vi "CODCr质控流程 (子VI).vi"(10 "CODCr量程切换":enum32{"H", "L", "AUTO"}(ring)=enum."AUTO", 11 "CODCr":bool) -> (2 "CODCr中断报警":bool, 3 "布尔":bool)   [LabVIEW 2016, in "质控单元.lvlib"]
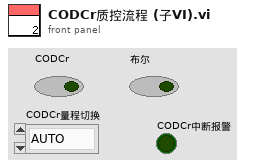
[diagram p1: front panel]
types:
  T1 = enum16{"待机", "启动水样测量", "水样测量中", "启动加标", "启动加标回收", "加标回收测量中", "结束"}
  T2 = cluster{"测量模式":enum16{"水样测量", "标样核查", "零点核查", "跨度核查", "空白测试", "加标回收", "平行样", "校零", "校标"}}
  T3 = enum16{"空闲", "水样测试", "标样核查", "零点核查", "跨度核查", "空白测试", "平行样测试", "加标回收", "空白校准", "标样校准", "初始化（清洗）"}
  T4 = cluster{"系统时间":timestamp, "工作状态":enum16{"空闲", "水样测试", "标样核查", "零点核查", "跨度核查", "空白测试", "平行样测试", "加标回收", "空白校准", "标样校准", "初始化（清洗）"}, "测量模式":enum16{"待机", "连续模式", "周期模式", "定点模式", "受控模式", "手动模式"}, "告警代码":enum16{"无告警", "缺试剂告警", "缺水样告警", "缺蒸馏水告警", "缺标液告警", "仪表漏液告警", "标定异常告警", "超量程告警", "加热异常", "低试剂预警", "超上限告警", "超下限告警", "仪表内部其他异常", "滴定异常告警", "电极异常告警", "量程切换告警", "参数设置告警", "PH电极电位异常", "电导率电极异常", "浊度光度异常", "溶解氧电极异常", "溶解氧光强异常", "温度异常告警", "PH异常告警", "溶解氧异常告警", "电导率异常告警", "浊度异常告警", "叶绿素异常告警", "藻密度异常告警", "蓝绿藻异常告警", "ORP异常告警", "氨氮异常告警", "清洁刷异常告警", "SD卡异常告警", "蓝牙异常告警", "Wifi异常告警", "流程异常告警"}, "故障代码":enum16{"无故障", "电机故障", "温度故障", "通讯故障", "滴定故障"}, "日志代码":u16, "软件版本":u16, "F0":sgl, "F1":sgl, "F2":sgl, "F3":sgl, "T":sgl, "H":sgl, "id":u16, "flowid":u16, "量程":u16, "总磷控温温度1":sgl, "营养盐控温温度2":sgl, "ADC":sgl}
  T5 = cluster{"因子编码":u32, "单位":u16, "标样参考值":sgl, "水样数据时间":timestamp, "水样实测值":sgl, "水样数据标识":string, "标样数据时间":timestamp, "标样实测值":sgl, "标样数据标识":string, "空白数据时间":timestamp, "空白实测值":sgl, "空白数据标识":string, "零点核查数据时间":timestamp, "零点核查实测值":sgl, "零点核查数据标识":string, "跨度核查数据时间":timestamp, "跨度核查实测值":sgl, "跨度核查数据标识":string, "加标回收数据时间":timestamp, "加标回收实测值":sgl, "加标回收数据标识":string, "平行样数据时间":timestamp, "平行样实测值":sgl, "平行样数据标识":string}
  T6 = cluster{"量程":dbl, "检出限":dbl, "加标前水样浓度":dbl, "加标后水样浓度":dbl, "加标水杯定容体积":dbl, "加标母液浓度":dbl, "加标体积":dbl, "加标回收率":dbl}
  T7 = cluster{"氨氮":u8, "总磷":u8, "总氮":u8, "CODMn":u8, "CODCr":u8}
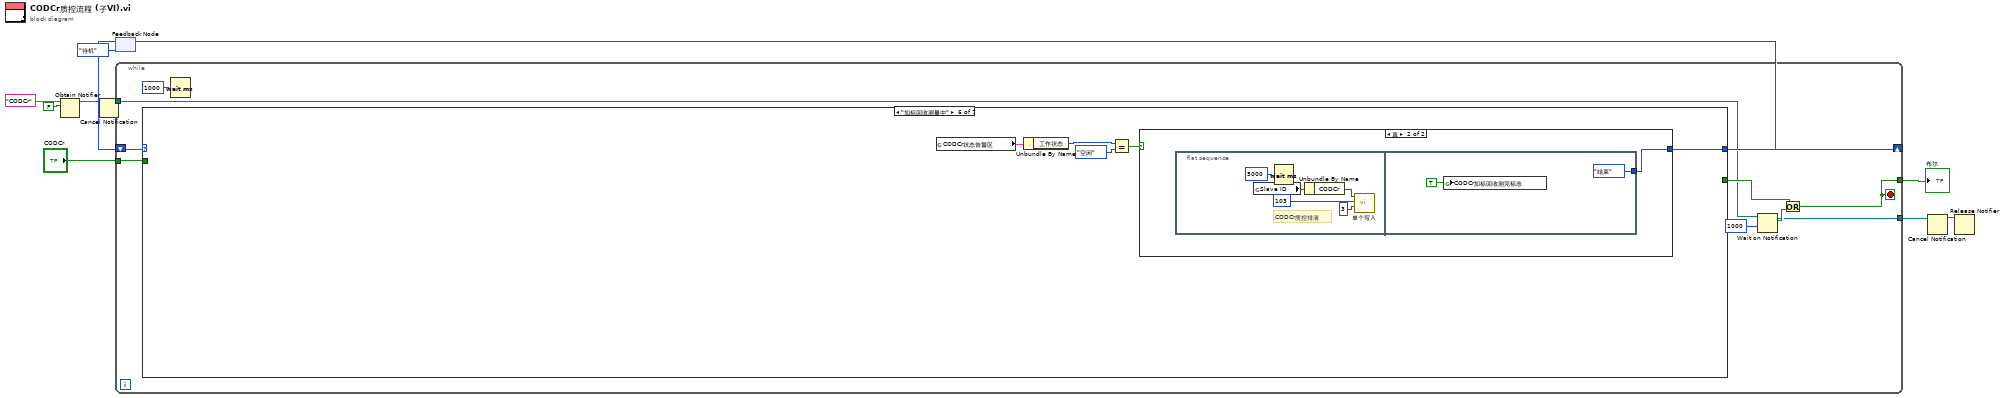
[diagram p0: block diagram]
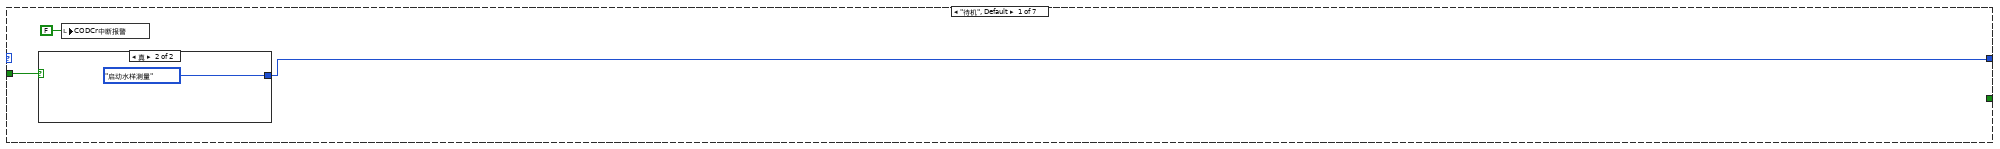
[diagram p2: hidden frame]
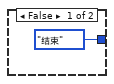
[diagram p3: hidden frame]
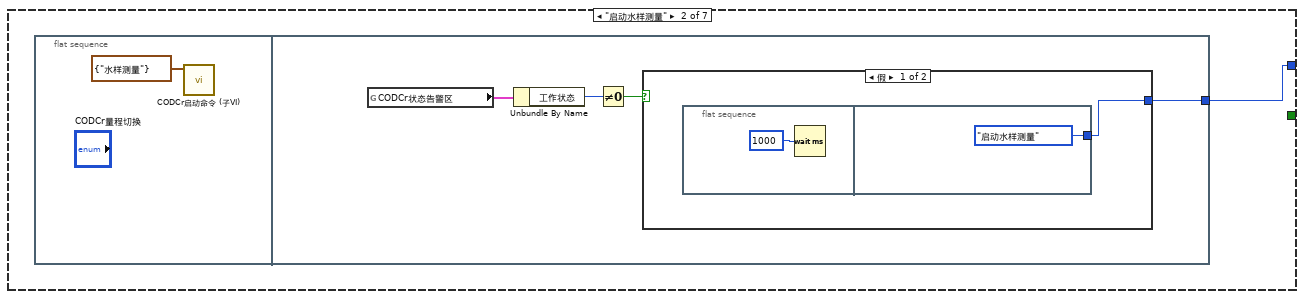
[diagram p4: hidden frame]
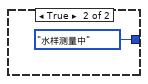
[diagram p5: hidden frame]
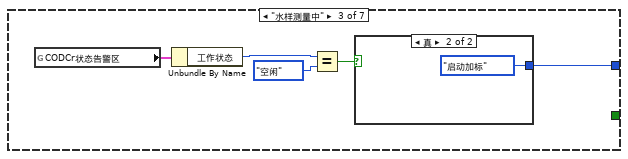
[diagram p6: hidden frame]
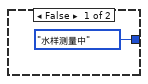
[diagram p7: hidden frame]
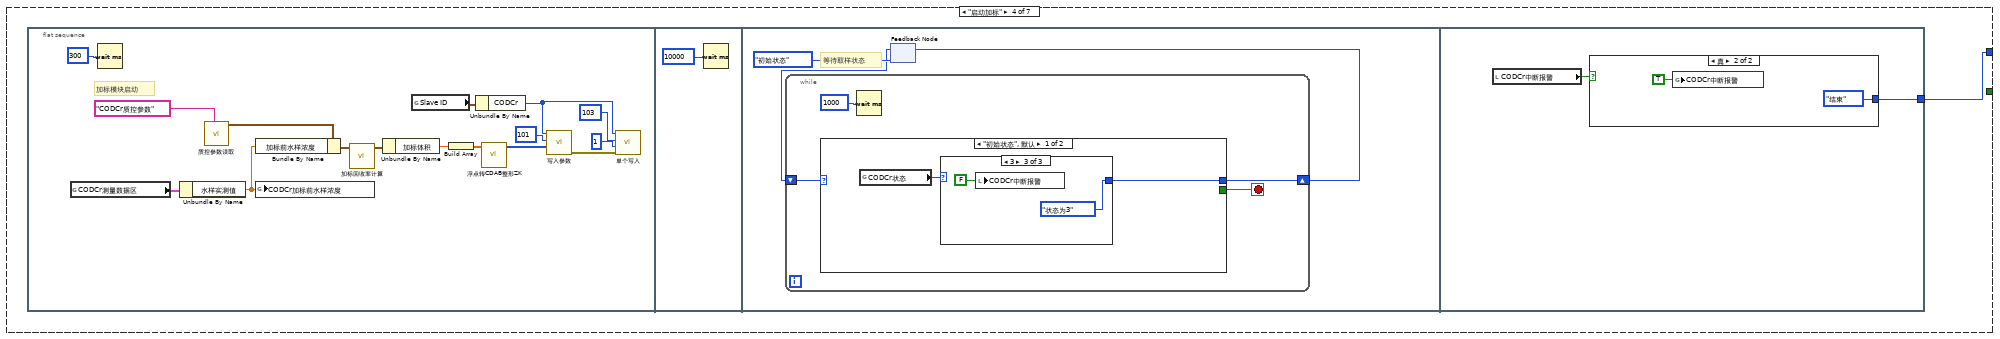
[diagram p8: hidden frame]
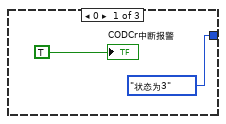
[diagram p9: hidden frame]
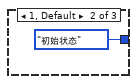
[diagram p10: hidden frame]
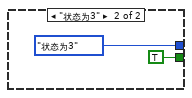
[diagram p11: hidden frame]
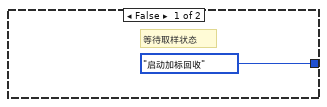
[diagram p12: hidden frame]
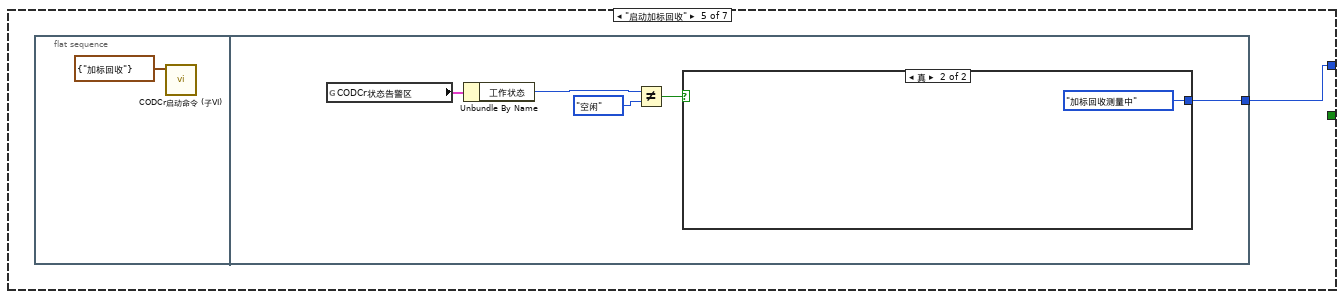
[diagram p13: hidden frame]
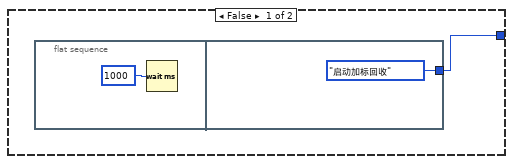
[diagram p14: hidden frame]
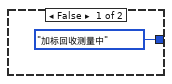
[diagram p15: hidden frame]
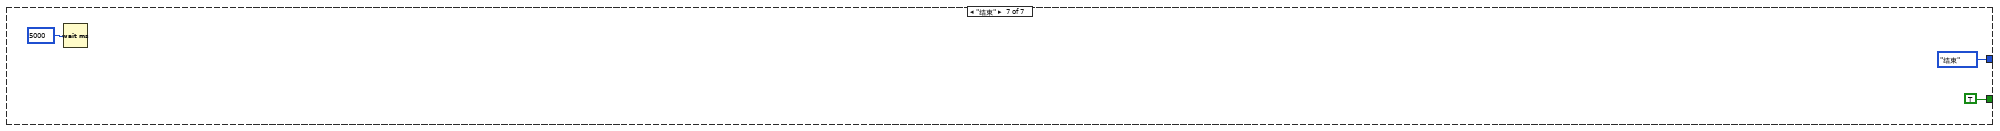
[diagram p16: hidden frame]
diagram:
  n1 = Obtain Notifier(name (unnamed)="CODCr" ("名称（未命名）"), notification data type=FALSE) -> (notifier out=w2:refnum<notifier>)  [unwired: 2 in, 2 out]
  n2 = Cancel Notification(0:w2) -> (8:w1:refnum<notifier>)  [unwired: 1 in, 2 out]
  n3 = feedback #1(T1."待机") -> (w7:T1)
  n4 = while {
    tunnel: "CODCr" -> [w21]
    tunnel: [w13] -> w9
    shift-right: [w20] -> w10
    shift-left: w7 -> [w18]
    tunnel: [w15] -> w3
    tunnel: w1 -> [w14]
    stop <- w13 stop-if-true
    n5 = case shown="\"加标回收测量中\"" w18 {
      tunnel: [w24 w27 w41 w44 w83 w98 T1."结束"] -> w20
      tunnel: [_ _ _ _ _ _ TRUE] -> w16
      tunnel: w21 -> [w23 _ _ _ _ _ _]
      frame "待机", Default {
        n6 = case shown="真" w23 {
          tunnel: [T1."结束" T1."启动水样测量"] -> w24
          frame False {
          }
          frame True {
          }
        }
        n7 = local write "CODCr中断报警"(FALSE ("CODMn中断报警")) -> ()
      }
      frame "启动水样测量" {
        n8 = flat-sequence {
          tunnel: [w32] -> w27
          frame #0 {
            n9 = call "CODCr启动命令 (子VI).vi"("启动测量模式"=T2 {"测量模式"=enum."水样测量"}) -> ()  [unwired: 10 in, 1 out]
          }
          frame #1 {
            n10 = global read "与CODCr交互全局.vi" "CODCr状态告警区"() -> (w30:T4)
            n11 = Unbundle By Name(w30) -> ("工作状态"=w31:T3)
            n12 = Not Equal To 0?(x=w31) -> (x != 0?=w29:bool)
            n13 = case shown="假" w29 {
              tunnel: [w33 T1."水样测量中"] -> w32
              frame False {
                n14 = flat-sequence {
                  tunnel: [T1."启动水样测量"] -> w33
                  frame #0 {
                    n15 = Wait (ms)(milliseconds to wait=u32 1000 ("等待时间（毫秒）")) -> ()  [unwired: 1 out]
                  }
                  frame #1 {
                  }
                }
              }
              frame True {
              }
            }
          }
        }
      }
      frame "水样测量中" {
        n16 = global read "与CODCr交互全局.vi" "CODCr状态告警区"() -> (w38:T4)
        n17 = Unbundle By Name(w38) -> ("工作状态"=w37:T3)
        n18 = Equal?(x=w37, y=T3."空闲") -> (x = y?=w39:bool)
        n19 = case shown="真" w39 {
          tunnel: [T1."水样测量中" T1."启动加标"] -> w41
          frame False {
          }
          frame True {
          }
        }
      }
      frame "启动加标" {
        n20 = flat-sequence {
          tunnel: [w79] -> w44
          frame #0 {
            # "加标模块启动"
            n21 = global read "与CODCr交互全局.vi" "CODCr测量数据区"() -> (w47:T5)
            n22 = Wait (ms)(milliseconds to wait=u32 300 ("等待时间（毫秒）")) -> ()  [unwired: 1 out]
            n23 = Unbundle By Name(w47) -> ("水样实测值"=w48:sgl)
            n24 = call "质控参数读取.vi"("section"="CODCr质控参数") -> ("参数"=w58:T6)  [unwired: 9 in, 1 out]
            n25 = Bundle By Name(cluster=w58, "加标前水样浓度"=w48) -> (w59:T6)
            n26 = global write "水样浓度全局.vi" "CODCr加标前水样浓度"(w48) -> ()
            n27 = call "加标回收率计算.vi"("参数"=w59) -> ("参数 out"=w57:T6)  [unwired: 9 in, 1 out]
            n28 = Unbundle By Name(w57) -> ("加标体积"=w50:dbl)
            n29 = global read "断电保存全局.vi" "Slave ID"() -> (w46:T7)
            n30 = Build Array(w50) -> (w56:dbl[])
            n31 = Unbundle By Name(w46) -> ("CODCr"=w45:u8)
            n32 = call "浮点转CDAB整形ZK.vi"("浮点数"=w56) -> ("CDAB整形输出"=w51:u16[])  [unwired: 10 in]
            n33 = call "写入参数.vi"("values"=w51, "starting address"=u16 101, "Slave ID"=w45) -> ("error out"=w55:errorcluster)  [unwired: 8 in]
            n34 = call "单个写入.vi"("Error in"=w55, "value"=u16 1, "address"=u16 103, "Slave ID"=w45) -> ()  [unwired: 7 in, 1 out]
          }
          frame #1 {
            n35 = Wait (ms)(milliseconds to wait=u32 10000 ("等待时间（毫秒）")) -> ()  [unwired: 1 out]
          }
          frame #2 {
            # "等待取样状态"
            n36 = feedback #2(enum16{"初始状态", "状态为3"}."初始状态") -> (w63:enum16{"初始状态", "状态为3"})
            n37 = while {
              shift-right: [w67] -> w62
              shift-left: w63 -> [w68]
              stop <- w66 stop-if-true
              n38 = case shown="\"初始状态\", 默认" w68 {
                tunnel: [w70 enum16{"初始状态", "状态为3"}."状态为3"] -> w67
                tunnel: [_ TRUE] -> w66
                frame "初始状态", Default {
                  n39 = global read "加标回收状态全局变量.vi" "CODCr状态"() -> (w69:u16)
                  n40 = case shown="3" w69 {
                    tunnel: [enum16{"初始状态", "状态为3"}."状态为3" enum16{"初始状态", "状态为3"}."初始状态" enum16{"初始状态", "状态为3"}."状态为3"] -> w70
                    frame 0 {
                      "CODCr中断报警" <- TRUE ("CODMn中断报警")
                    }
                    frame 1, Default {
                    }
                    frame 3 {
                      n41 = local write "CODCr中断报警"(FALSE ("CODMn中断报警")) -> ()
                    }
                  }
                }
                frame "状态为3" {
                }
              }
              n42 = Wait (ms)(milliseconds to wait=u32 1000 ("等待时间（毫秒）")) -> ()  [unwired: 1 out]
            }
            n43 = feedback-in #2(w62) -> ()
          }
          frame #3 {
            n44 = local read "CODCr中断报警"() -> (w78:bool)
            n45 = case shown="真" w78 {
              tunnel: [T1."启动加标回收" T1."结束"] -> w79
              frame False {
                # "等待取样状态"
              }
              frame True {
                n46 = global write "质控中断报警全局.vi" "CODCr中断报警"(TRUE ("CODCr中断报警")) -> ()
              }
            }
          }
        }
      }
      frame "启动加标回收" {
        n47 = flat-sequence {
          tunnel: [w89] -> w83
          frame #0 {
            n48 = call "CODCr启动命令 (子VI).vi"("启动测量模式"=T2 {"测量模式"=enum."加标回收"}) -> ()  [unwired: 10 in, 1 out]
          }
          frame #1 {
            n49 = global read "与CODCr交互全局.vi" "CODCr状态告警区"() -> (w88:T4)
            n50 = Unbundle By Name(w88) -> ("工作状态"=w87:T3)
            n51 = Not Equal?(x=w87, y=T3."空闲") -> (x != y?=w85:bool)
            n52 = case shown="真" w85 {
              tunnel: [w90 T1."加标回收测量中"] -> w89
              frame False {
                n53 = flat-sequence {
                  tunnel: [T1."启动加标回收"] -> w90
                  frame #0 {
                    n54 = Wait (ms)(milliseconds to wait=u32 1000 ("等待时间（毫秒）")) -> ()  [unwired: 1 out]
                  }
                  frame #1 {
                  }
                }
              }
              frame True {
              }
            }
          }
        }
      }
      frame "加标回收测量中" {
        n55 = global read "与CODCr交互全局.vi" "CODCr状态告警区"() -> (w95:T4)
        n56 = Unbundle By Name(w95) -> ("工作状态"=w94:T3)
        n57 = Equal?(x=w94, y=T3."空闲") -> (x = y?=w96:bool)
        n58 = case shown="真" w96 {
          tunnel: [T1."加标回收测量中" w100] -> w98
          frame False {
          }
          frame True {
            n59 = flat-sequence {
              tunnel: [T1."结束"] -> w100
              frame #0 {
                # "CODCr质控排液"
                n60 = global read "断电保存全局.vi" "Slave ID"() -> (w102:T7)
                n61 = Wait (ms)(milliseconds to wait=u32 5000 ("等待时间（毫秒）")) -> ()  [unwired: 1 out]
                n62 = Unbundle By Name(w102) -> ("CODCr"=w101:u8)
                n63 = call "单个写入.vi"("value"=u16 3, "address"=u16 103, "Slave ID"=w101) -> ()  [unwired: 8 in, 1 out]
              }
              frame #1 {
                n64 = global write "质控测完标志全局 1.vi" "CODCr加标回收测完标志"(TRUE ("COD加标回收测完标志")) -> ()
              }
            }
          }
        }
      }
      frame "结束" {
        n65 = Wait (ms)(milliseconds to wait=u32 5000 ("等待时间（毫秒）")) -> ()  [unwired: 1 out]
      }
    }
    n66 = Wait (ms)(milliseconds to wait=u32 1000 ("等待时间（毫秒）")) -> ()  [unwired: 1 out]
    n67 = Wait on Notification(notifier=w14, timeout in ms (-1)=1000 ("超时毫秒(-1)")) -> (notifier out=w15:refnum<notifier>, notification=w17:bool)  [unwired: 2 in, 2 out]
    n68 = Or(x=w16, y=w17) -> (x .or. y?=w13:bool)
  }
  "布尔" <- w9
  n69 = feedback-in #1(w10) -> ()
  n70 = Cancel Notification(0:w3) -> (8:w4:refnum<notifier>)  [unwired: 1 in, 2 out]
  n71 = Release Notifier(notifier=w4) -> ()  [unwired: 2 in, 3 out]
